vi "Auto Inputs.vi"(8 "error in":errorcluster) -> (0 "error out":errorcluster, 1 "Auto Notifiers Out":T17, 3 "Auto Refs":T1={"Ultrasonic Forward"={"AIDeviceRef"={"DevStatus"={"status"=FALSE, "code"=0, "source"=""}, "Controller"=enum."Controller 1", "Analog Channel"=enum."Invalid"}, "Scaling factor (V/in)"=0.0098, "Average Bits"=3}, "Ultrasonic Back"={"AIDeviceRef"={"DevStatus"={"status"=FALSE, "code"=0, "source"=""}, "Controller"=enum."Controller 1", "Analog Channel"=enum."Invalid"}, "Scaling factor (V/in)"=0.0098, "Average Bits"=3}, "Strafe Motor"={"DeviceStatus"={"status"=FALSE, "code"=0, "source"=""}, "Type"=enum."PWM", "PWM"={"Controller"=enum."Controller 1", "PWM Channel"=enum."PWM 0", "DeadBand"={"Name"="", "maxPositivePwm"=0, "minPositivePwm"=0, "centerPwm"=0, "maxNegativePwm"=0, "minNegativePwm"=0, "angularRange"=0}}, "CAN"={"Device Number"=0, "Control Mode"=enum."Percent VBus", "Semaphore"=refnum, "Max Vout"=0.0, "TalonSRX Control Mode"=enum."Percent VBus"}, "Invert"=FALSE, "TransformRef"=refnum, "InvTransformRef"=refnum}, "Drive Motors"={"DevStatus"={"status"=FALSE, "code"=0, "source"=""}, "Motors[]"=[], "Square Inputs"=FALSE, "Max Output"=0.0}, "Gyro"={"DevStatus"={"status"=FALSE, "code"=0, "source"=""}, "Analog Module"=enum."Controller 1", "Analog Channel"=enum."Invalid", "Offset"=0.0, "Gain (VoltsPerDegree/Second)"=0.0}} {"Ultrasonic Back"."Average Bits" max=15; "Ultrasonic Forward"."Average Bits" max=15})   [LabVIEW 2014]
uses:
  Auto Notifiers.ctl
  Main/Arms/Arm clapper state.ctl
  Main/Arms/Arm State.ctl
  Auto Refs.ctl
  <vilib>/Rock Robotics/WPI/Ultrasonic/WPI_SonarMB1010AnalogDeviceRef.ctl
  <vilib>/Rock Robotics/WPI/AnalogChannel/WPI_AnalogChannelDevRef.ctl
  <vilib>/Rock Robotics/SystemInterfaces/Typedef/FPGA_TypedefAnalogModule.ctl
  <vilib>/Rock Robotics/SystemInterfaces/AI/FPGA_AIChannel.ctl
  <vilib>/Rock Robotics/WPI/MotorControl/WPI_MotorControlDeviceRef.ctl
  <vilib>/Rock Robotics/WPI/MotorControl/WPI_MotorControlType.ctl
  <vilib>/Rock Robotics/SystemInterfaces/Typedef/FPGA_TypedefDigitalModule.ctl
  <vilib>/Rock Robotics/SystemInterfaces/DIO/FPGA_DIOPWMChannel.ctl
  <vilib>/Rock Robotics/WPI/PWM/WPI_PWMDeadband.ctl
  <vilib>/Rock Robotics/WPI/CAN/Jaguar/SubVIs/WPI_CANJaguar_ControlMode.ctl
  <vilib>/Rock Robotics/WPI/CAN/TalonSRX/WPI_CANTalonSRX_APIControlMode.ctl
  <vilib>/Rock Robotics/WPI/PWM/WPI_PWMTransform_ConPane.ctl
  <vilib>/Rock Robotics/WPI/RobotDrive/WPI_RobotDriveDevRef.ctl
  <vilib>/Rock Robotics/WPI/Gyro/WPI_GyroDevRef.ctl
  Utilities/Sensor Refname.ctl
  Utilities/Refname.ctl
  Utilities/Sensor Refname to String.vi
  Utilities/RefnameToString.vi
  <vilib>/Rock Robotics/WPI/Ultrasonic/WPI_SonarMB1010AnalogRefNum Registry Get.vi
  <vilib>/Rock Robotics/WPI/RobotDrive/WPI_RobotDriveGetSetRefNum.vi
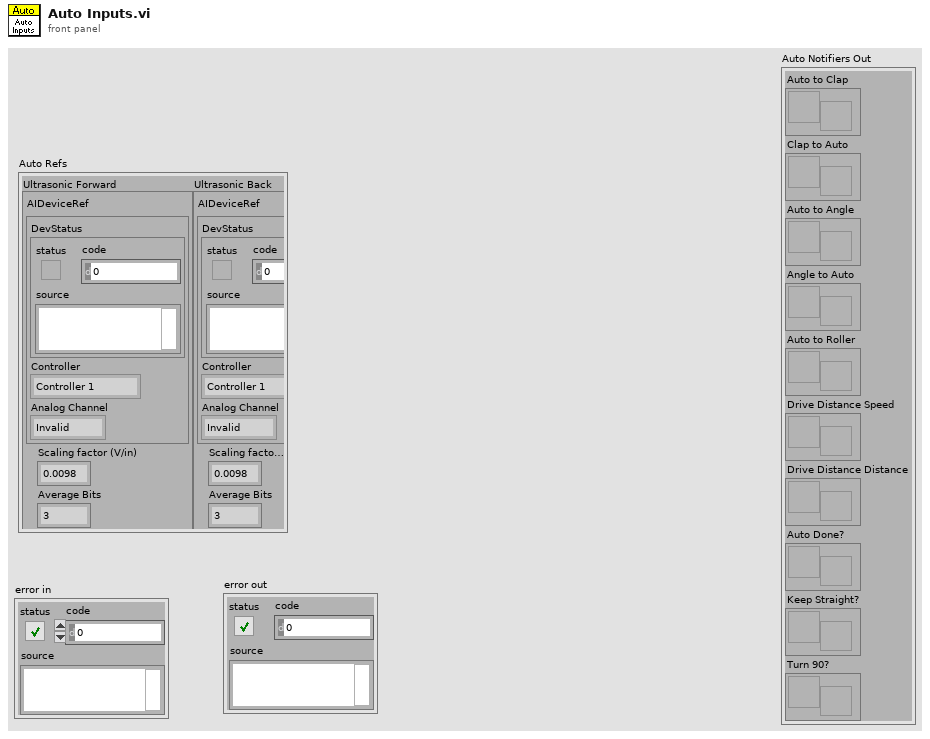
[diagram p1: front panel]
types:
  T1 = typedef "Auto Refs.ctl" = cluster{"Ultrasonic Forward":T2, "Ultrasonic Back":T2, "Strafe Motor":T6, "Drive Motors":T15, "Gyro":T16}
  T2 = typedef "WPI_SonarMB1010AnalogDeviceRef.ctl" = cluster{"AIDeviceRef":T3, "Scaling factor (V/in)":dbl, "Average Bits":u8}
  T3 = typedef "WPI_AnalogChannelDevRef.ctl" = cluster{"DevStatus":errorcluster, "Controller":T4, "Analog Channel":T5}
  T4 = typedef "FPGA_TypedefAnalogModule.ctl" = enum16{"Controller 1"}
  T5 = typedef "FPGA_AIChannel.ctl" = enum8{"AI 0", "AI 1", "AI 2", "AI 3", "AI MXP 0", "AI MXP 1", "AI MXP 2", "AI MXP 3", "Invalid"}
  T6 = typedef "WPI_MotorControlDeviceRef.ctl" = cluster{"DeviceStatus":errorcluster, "Type":T7, "PWM":cluster{"Controller":T8, "PWM Channel":T9, "DeadBand":T10}, "CAN":cluster{"Device Number":u8, "Control Mode":T11, "Semaphore":T12, "Max Vout":dbl, "TalonSRX Control Mode":T13}, "Invert":bool, "TransformRef":T14, "InvTransformRef":T14}
  T7 = typedef "WPI_MotorControlType.ctl" = enum16{"PWM", "CAN", "CANTalonSRX"}
  T8 = typedef "FPGA_TypedefDigitalModule.ctl" = enum16{"Controller 1"}
  T9 = typedef "FPGA_DIOPWMChannel.ctl" = enum8{"PWM 0", "PWM 1", "PWM 2", "PWM 3", "PWM 4", "PWM 5", "PWM 6", "PWM 7", "PWM 8", "PWM 9", "PWM MXP 0", "PWM MXP 1", "PWM MXP 2", "PWM MXP 3", "PWM MXP 4", "PWM MXP 5", "PWM MXP 6", "PWM MXP 7", "PWM MXP 8", "PWM MXP 9", "Invalid"}
  T10 = typedef "WPI_PWMDeadband.ctl" = cluster{"Name":string, "maxPositivePwm":i32, "minPositivePwm":i32, "centerPwm":i32, "maxNegativePwm":i32, "minNegativePwm":i32, "angularRange":u16}
  T11 = typedef "WPI_CANJaguar_ControlMode.ctl" = enum8{"Percent VBus", "Current", "Speed", "Position", "Voltage"}
  T12 = typedef "Semaphore RefNum" = refnum<k1>
  T13 = typedef "WPI_CANTalonSRX_APIControlMode.ctl" = enum8{"Percent VBus", "Speed", "Position", "Slave", "Unchanged / Invalid"}
  T14 = typedef "WPI_PWMTransform_ConPane.ctl" = refnum<vi>
  T15 = typedef "WPI_RobotDriveDevRef.ctl" = cluster{"DevStatus":errorcluster, "Motors[]":T6[], "Square Inputs":bool, "Max Output":dbl}
  T16 = typedef "WPI_GyroDevRef.ctl" = cluster{"DevStatus":errorcluster, "Analog Module":T4, "Analog Channel":T5, "Offset":dbl, "Gain (VoltsPerDegree/Second)":dbl}
  T17 = typedef "Auto Notifiers.ctl" = cluster{"Auto to Clap":refnum<notifier>, "Clap to Auto":refnum<notifier>, "Auto to Angle":refnum<notifier>, "Angle to Auto":refnum<notifier>, "Auto to Roller":refnum<notifier>, "Drive Distance Speed":refnum<notifier>, "Drive Distance Distance":refnum<notifier>, "Auto Done?":refnum<notifier>, "Keep Straight?":refnum<notifier>, "Turn 90?":refnum<notifier>}
  T18 = typedef "Sensor Refname.ctl" = enum16{"Gyro", "Elevator Top LS", "Elevator Bottom LS", "Claw Outside LS", "Left Drive Encoder", "Right Drive Encoder", "Strafe Encoder", "Elevator Encoder", "Ultrasonic Forward", "Ultrasonic Back", "Arm Angle POT", "Arm Clapper POT", "Accelerometer", "Tote LS", "DIP 1", "DIP 2", "DIP 3", "DIP 4"}
  T19 = typedef "Arm clapper state.ctl" = enum16{"In", "Tote Closed", "Bin Closed", "Straight", "Open"}
  T20 = typedef "Arm State.ctl" = enum16{"Ground", "Level", "Feeder", "Vertical"}
  T21 = typedef "Refname.ctl" = enum16{"Gamepad 1", "Gamepad 2", "Drive Motors", "Strafe Motor", "Arm Clapper Motor", "Arm Angle", "Arm Belt Left", "Arm Belt Right", "Elevator 1", "Elevator 2", "Wiper"}
  T22 = cluster{"SonarMB1010AnalogDevRef":T2, "SonarMB1010AnalogDevRef":T2, "MotorControlDevRef":T6, "RobotDriveDevRef":T15, "GyroDevRef":T16}
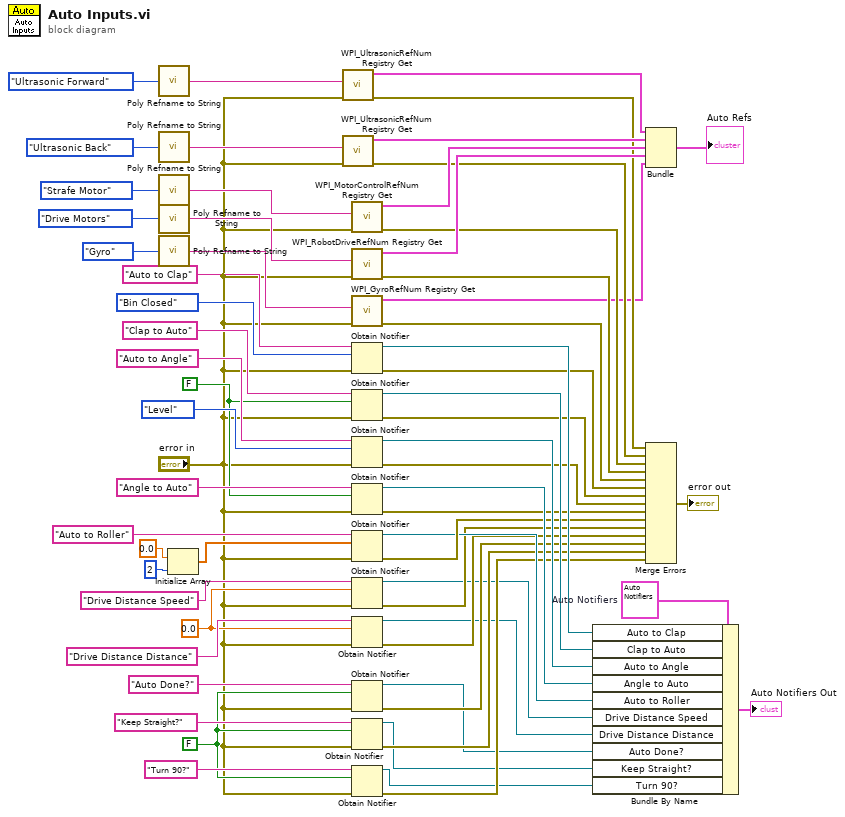
[diagram p0: block diagram]
diagram:
  w4 = T17 {"Auto to Clap"=refnum, "Clap to Auto"=refnum, "Auto to Angle"=refnum, "Angle to Auto"=refnum, "Auto to Roller"=refnum, "Drive Distance Speed"=refnum, "Drive Distance Distance"=refnum, "Auto Done?"=refnum, "Keep Straight?"=refnum, "Turn 90?"=refnum}  # Auto Notifiers
  w16 = FALSE
  w17 = 0.0
  w30 = FALSE
  n1 = call-poly "Poly Refname to String.vi"("Sensor Refnames"=Sensor_Refname."Ultrasonic Forward" ("Sensor Refname")) -> ("Refname"=w63:string)
  n2 = call-poly "Poly Refname to String.vi"("Sensor Refnames"=Sensor_Refname."Ultrasonic Back" ("Sensor Refname")) -> ("Refname"=w61:string)
  n3 = call-poly "Poly Refname to String.vi"("Enum"=Refname."Strafe Motor" ("Refname")) -> ("Refname"=w59:string)
  n4 = call-poly "Poly Refname to String.vi"("Enum"=Refname."Drive Motors" ("Refname")) -> ("Refname"=w57:string)
  n5 = call-poly "Poly Refname to String.vi"("Sensor Refnames"=Sensor_Refname."Gyro" ("Sensor Refname")) -> ("Refname"=w50:string)
  n6 = Initialize Array(0.0 ("element"), 2 ("dimension size")) -> (w26:dbl[])
  n7 = call-poly <vilib>:"WPI_UltrasonicRefNum Registry Get.vi"("error in (no error)"="error in", "refnum name"=w63) -> ("error out"=w46:errorcluster, "SonarMB1010AnalogDevRef"=w45:T2)  [unwired: 8 in]
  n8 = call-poly <vilib>:"WPI_UltrasonicRefNum Registry Get.vi"("error in (no error)"="error in", "refnum name"=w61) -> ("error out"=w47:errorcluster, "SonarMB1010AnalogDevRef"=w48:T2)  [unwired: 8 in]
  n9 = call <vilib>:"WPI_MotorControlRefNum Registry Get.vi"("error in (no error)"="error in", "refnum name"=w59) -> ("error out"=w54:errorcluster, "MotorControlDevRef"=w56:T6)  [unwired: 8 in]
  n10 = call <vilib>:"WPI_RobotDriveRefNum Registry Get.vi"("error in (no error)"="error in", "refnum name"=w57) -> ("error out"=w53:errorcluster, "RobotDriveDevRef"=w55:T15)  [unwired: 8 in]
  n11 = call <vilib>:"WPI_GyroRefNum Registry Get.vi"("error in (no error)"="error in", "refnum name"=w50) -> ("error out"=w49:errorcluster, "GyroDevRef"=w1:T16)  [unwired: 8 in]
  n12 = Obtain Notifier(name (unnamed)="Auto to Clap", notification data type=Arm_clapper_state."Bin Closed" ("Enum"), error in (no error)="error in") -> (notifier out=w40:refnum<notifier>, error out=w36:errorcluster)  [unwired: 1 in, 1 out]
  n13 = Obtain Notifier(name (unnamed)="Clap to Auto", notification data type=w30, error in (no error)="error in") -> (notifier out=w39:refnum<notifier>, error out=w35:errorcluster)  [unwired: 1 in, 1 out]
  n14 = Obtain Notifier(name (unnamed)="Auto to Angle", notification data type=Arm_State."Level" ("Enum"), error in (no error)="error in") -> (notifier out=w38:refnum<notifier>, error out=w34:errorcluster)  [unwired: 1 in, 1 out]
  n15 = Obtain Notifier(name (unnamed)="Angle to Auto", notification data type=w30, error in (no error)="error in") -> (notifier out=w37:refnum<notifier>, error out=w33:errorcluster)  [unwired: 1 in, 1 out]
  n16 = Obtain Notifier(name (unnamed)="Auto to Roller", notification data type=w26, error in (no error)="error in") -> (notifier out=w23:refnum<notifier>, error out=w27:errorcluster)  [unwired: 1 in, 1 out]
  n17 = Obtain Notifier(name (unnamed)="Drive Distance Speed", notification data type=w17, error in (no error)="error in") -> (notifier out=w5:refnum<notifier>, error out=w14:errorcluster)  [unwired: 1 in, 1 out]
  n18 = Obtain Notifier(name (unnamed)="Drive Distance Distance", notification data type=w17, error in (no error)="error in") -> (notifier out=w9:refnum<notifier>, error out=w13:errorcluster)  [unwired: 1 in, 1 out]
  n19 = Obtain Notifier(name (unnamed)="Auto Done?", notification data type=w16, error in (no error)="error in") -> (notifier out=w8:refnum<notifier>, error out=w12:errorcluster)  [unwired: 1 in, 1 out]
  n20 = Obtain Notifier(name (unnamed)="Keep Straight?", notification data type=w16, error in (no error)="error in") -> (notifier out=w7:refnum<notifier>, error out=w11:errorcluster)  [unwired: 1 in, 1 out]
  n21 = Obtain Notifier(name (unnamed)="Turn 90?", notification data type=w16, error in (no error)="error in") -> (notifier out=w6:refnum<notifier>, error out=w10:errorcluster)  [unwired: 1 in, 1 out]
  n22 = Bundle By Name(cluster=w4, "Auto to Clap"=w40, "Clap to Auto"=w39, "Auto to Angle"=w38, "Angle to Auto"=w37, "Auto to Roller"=w23, "Drive Distance Speed"=w5, "Drive Distance Distance"=w9, "Auto Done?"=w8, "Keep Straight?"=w7, "Turn 90?"=w6) -> (→"Auto Notifiers Out":T17)
  n23 = Bundle("SonarMB1010AnalogDevRef"=w45, "SonarMB1010AnalogDevRef"=w48, "MotorControlDevRef"=w56, "RobotDriveDevRef"=w55, "GyroDevRef"=w1) -> (→"Auto Refs":T22)  [unwired: 1 in]
  n24 = Merge Errors(w46, w47, w54, w53, w49, w36, w35, w34, w33, w27, w14, w13, w12, w11, w10) -> (→"error out":errorcluster)
